vi "Split Version String.vi"(11 "version":string) -> (3 "split version":i32[](array[numeric]))   [LabVIEW 2015]
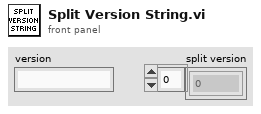
[diagram p1: front panel]
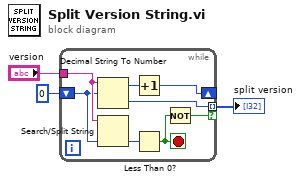
[diagram p0: block diagram]
diagram:
  n1 = while {
    tunnel: "version" -> [w10]
    shift-right: [w6] -> _
    shift-left: 0 -> [w9]
    tunnel: [w11] -> w3 mode=indexing if=w5
    stop <- w4 stop-if-true
    n2 = Decimal String To Number(string=w10, offset=w9) -> (offset past number=w7:i32, number=w11:i32)  [unwired: 1 in]
    n3 = Search/Split String(string=w10, offset (0)=w9) -> (offset of match=w8:i32)  [unwired: 1 in, 2 out]
    n4 = Increment(x=w7) -> (x+1=w6:i32)
    n5 = Less Than 0?(x=w8) -> (x < 0?=w4:bool)
    n6 = Not(x=w4) -> (.not. x?=w5:bool)
  }
  "split version" <- w3
